vi "if_v0_v0.vi"() -> ()   [LabVIEW 2009]
panel:
  out "Starea apei":string="Apa  lichida"
  in  "Temperatura":dbl(slide)=34.584717607973424 scale=-30.0..50.0
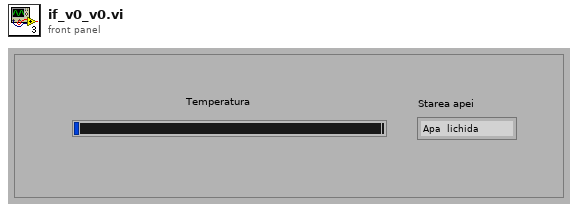
[diagram p1: front panel]
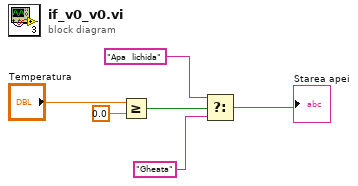
[diagram p0: block diagram]
diagram:
  n1 = Greater Or Equal?(x="Temperatura", y=0.0) -> (x >= y?=w4:bool)
  n2 = Select(t="Apa  lichida" ("Apa este lichida"), s=w4, f="Gheata") -> (s? t:f=→"Starea apei":string)
